vi "disconnect.vi"(8 "error in (no error)":errorcluster, 11 "TCPClient in":refnum<class "TCPClient.lvclass">) -> (0 "error out":errorcluster, 3 "TCPClient out":refnum<class "TCPClient.lvclass">)   [LabVIEW 2016, in "TCPClient.lvclass"]
uses:
  TCPClient.lvclass
  home/harini/tcs/ts_AtSpectrograph/ss_SpectrographInstrument/ts_labview_tcp/TCPCommunicator/TCPCommunicator.lvclass
  TCPCommunicator/TCPCommunicator.lvclass/TCPCommunicator.ctl
  TCPCommunicator/TCPCommunicator.lvclass
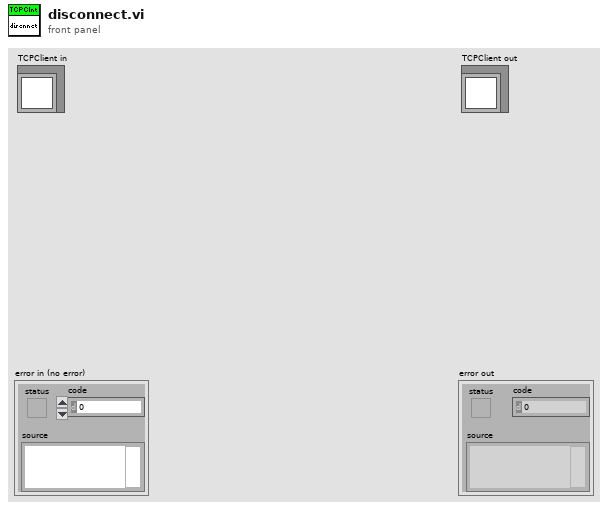
[diagram p1: front panel]
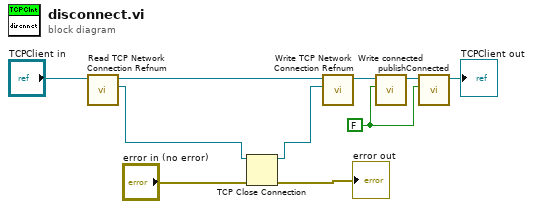
[diagram p0: block diagram]
diagram:
  w3 = FALSE ("connected")
  n1 = call-dynamic "Read TCP Network Connection Refnum.vi"("TCPCommunicator in"="TCPClient in") -> ("TCP Network Connection Refnum"=w10:refnum<k5>, "TCPCommunicator out"=w9:refnum<class "TCPClient.lvclass">)  [unwired: 8 in, 1 out]
  n2 = TCP Close Connection(connection ID=w10, error in (no error)="error in (no error)") -> (connection ID out=w8:refnum<k5>, error out=→"error out":errorcluster)  [unwired: 1 out]
  n3 = call-dynamic "Write TCP Network Connection Refnum.vi"("TCP Network Connection Refnum"=w8, "TCPCommunicator in"=w9) -> ("TCPCommunicator out"=w7:refnum<class "TCPClient.lvclass">)  [unwired: 8 in, 1 out]
  n4 = call "Write connected.vi"("connected"=w3, "TCPCommunicator in"=w7) -> ("TCPCommunicator out"=w4:refnum<class "TCPClient.lvclass">)  [unwired: 8 in, 1 out]
  n5 = call-dynamic "publishConnected.vi"("Connected"=w3, "TCPCommunicator in"=w4) -> ("TCPCommunicator out"=→"TCPClient out":refnum<class "TCPClient.lvclass">)  [unwired: 8 in, 1 out]
